vi "close.vi"(8 "error in (no error)":errorcluster, 11 "RobotIO in":refnum<class "RobotIO.lvclass">) -> (0 "error out":errorcluster, 3 "RobotIO out":refnum<class "RobotIO.lvclass">)   [LabVIEW 2019, in "RobotIO.lvclass"]
uses:
  RobotIO.lvclass
  IOCard.lvclass
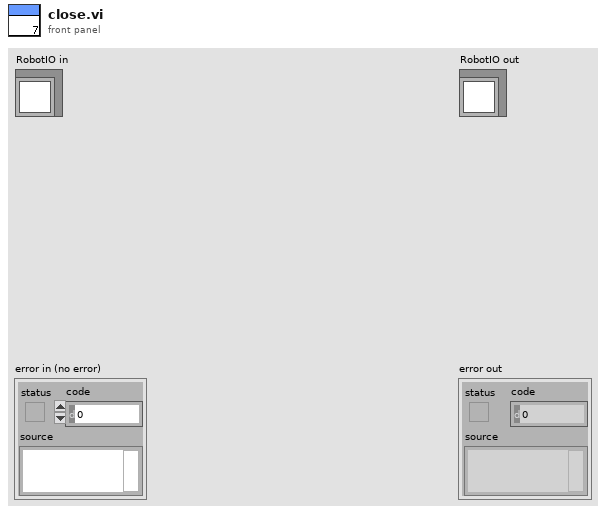
[diagram p1: front panel]
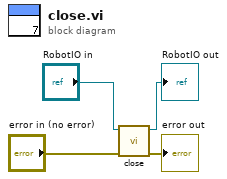
[diagram p0: block diagram]
diagram:
  n1 = call-parent "close.vi"("error in (no error)"="error in (no error)", "IOCard in"="RobotIO in") -> ("error out"=→"error out":errorcluster, "IOCard out"=→"RobotIO out":refnum<class "RobotIO.lvclass">)  [unwired: 8 in]
